vi "Write_comp_data.vi"(3 "error in":errorcluster, 4 "comp_data":T1(array[cluster]), 5 "ref in":i32) -> (0 "error out":errorcluster, 2 "ref out":i32)   [LabVIEW 2010]
uses:
  <vilib>/addons/h5labview2/base/hid_t.ctl
  <vilib>/addons/h5labview2/dataset/H5Dwrite.llb/H5Dwrite.xnode
  <vilib>/addons/h5labview2/base/lib_path.vi
  <vilib>/addons/h5labview2/base/H5Equery.vi
  <vilib>/addons/h5labview2/group/H5G.lvlib
  <vilib>/addons/h5labview2/attrib/H5A.lvlib
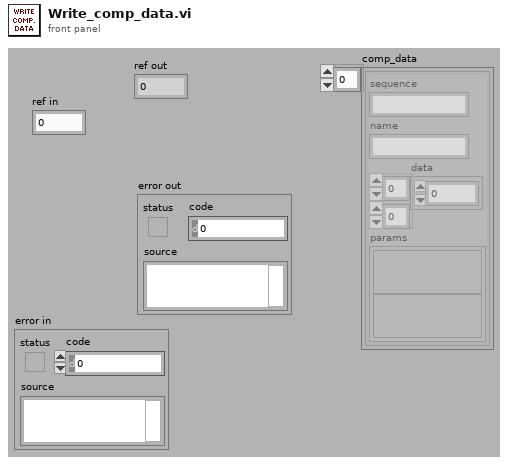
[diagram p1: front panel]
types:
  T1 = cluster{"sequence":string, "name":string, "data":sgl[][], "params":variant[]}[]
  T2 = typedef "hid_t.ctl" = i32
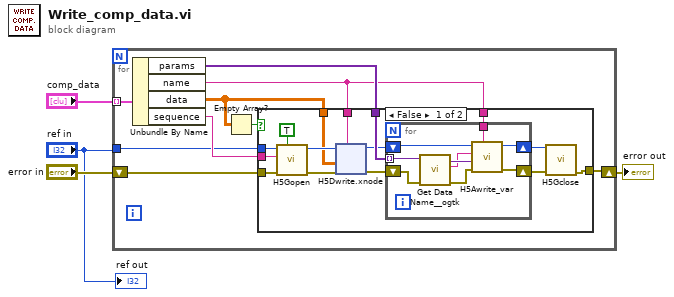
[diagram p0: block diagram]
diagram:
  n1 = for {
    tunnel: "comp_data" -> [w12] mode=indexing
    shift-right: [w8] -> w4
    shift-left: "error in" -> [w13]
    tunnel: "ref in" -> [w10]
    n2 = Unbundle By Name(w12) -> ("params"=w9:variant[], "name"=w5:string, "data"=w7:sgl[][], "sequence"=w11:string)
    n3 = Empty Array?(array=w7) -> (empty?=w6:bool)
    n4 = case shown="False" w6 {
      tunnel: w13 -> [w27 w56]
      tunnel: w11 -> [w26 _]
      tunnel: w10 -> [w28 _]
      tunnel: w9 -> [w20 _]
      tunnel: w5 -> [w24 _]
      tunnel: [w21 w56] -> w8
      tunnel: w7 -> [w23 _]
      tunnel: w5 -> [w14 _]
      frame False {
        n5 = call <vilib>:"H5Gopen.vi"("create? (F)"=TRUE ("Create if not found (F)"), "error in (no error)"=w27, "name"=w26, "ref in"=w28) -> ("error out"=w22:errorcluster, "group out"=w25:T2)  [unwired: 6 in]
        n6 = xnode "H5Dwrite.xnode"("dataset name"=w24, "error in (no error)"=w22, "data"=w23, "ref in"=w25) -> ("error out"=w18:errorcluster, "ref out"=w19:T2)  [unwired: 3 in, 1 out]
        n7 = for {
          tunnel: w20 -> [w33] mode=indexing
          shift-right: [w37] -> w17
          shift-left: w19 -> [w35]
          shift-right: [w36] -> w16
          shift-left: w18 -> [w30]
          tunnel: w14 -> [w34]
          n8 = call <userlib>:"Get Data Name__ogtk.vi"("error in (no error)"=w30, "Data"=w33) -> ("error out"=w29:errorcluster, "Data Name"=w31:string, "Data dup"=w32:variant)  [unwired: 7 in]
          n9 = call <vilib>:"H5Awrite_var.vi"("object name"=w34, "error in (no error)"=w29, "data"=w32, "attrib name"=w31, "ref in"=w35) -> ("error out"=w36:errorcluster, "ref out"=w37:T2)  [unwired: 4 in, 1 out]
        }
        n10 = call <vilib>:"H5Gclose.vi"("error in (no error)"=w16, "group in"=w17) -> ("error out"=w21:errorcluster)  [unwired: 9 in]
      }
      frame True {
      }
    }
  }
  "error out" <- w4
  "ref out" <- "ref in"
